vi "Version 1_Read Fullscale Values.vi"(7 "Address (A)":string="A", 8 "error in":errorcluster, 10 "Software version (optional - wire for speed)":u8, 11 "VISA Session In":refnum<visa-resource-name>="Alicat") -> (0 "error out":errorcluster, 1 "Signed?":T1, 2 "Fullscale":T2={"Pressure"=nan, "Volumetric"=nan, "Mass"=nan} {"Pressure" format="%_4f"; "Volumetric" format="%_4f"; "Mass" format="%_4f"}, 3 "VISA Session Out":refnum<visa-resource-name>)   [LabVIEW 2019]
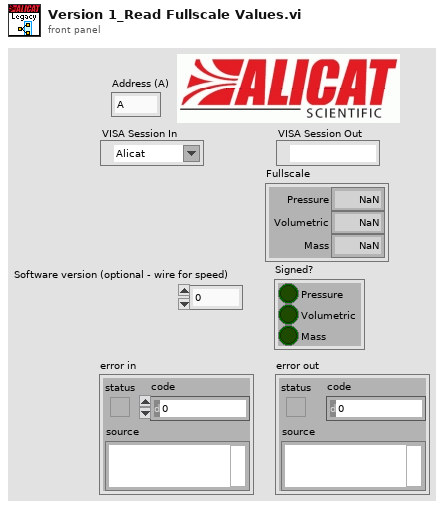
[diagram p1: front panel]
types:
  T1 = cluster{"Pressure":bool, "Volumetric":bool, "Mass":bool}
  T2 = cluster{"Pressure":dbl, "Volumetric":dbl, "Mass":dbl}
  T3 = cluster{"Absolute Pressure":dbl, "Gauge/Diff. Pressure":dbl, "Volumetric Flow":dbl, "Mass Flow":dbl}
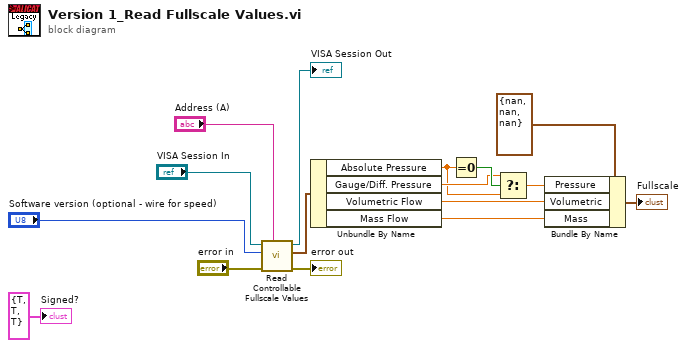
[diagram p0: block diagram]
diagram:
  n1 = call "Read Controllable Fullscale Values.vi"("Unit ID (A)"="Address (A)", "error in"="error in", "Software Version"="Software version (optional - wire for speed)", "VISA Session In"="VISA Session In") -> ("error out"=→"error out":errorcluster, "Fullscale"=w7:T3, "VISA Session Out"=→"VISA Session Out":refnum<visa-resource-name>)  [unwired: 5 in]
  n2 = Unbundle By Name(w7) -> ("Absolute Pressure"=w2:dbl, "Gauge/Diff. Pressure"=w3:dbl, "Volumetric Flow"=w6:dbl, "Mass Flow"=w5:dbl)
  n3 = Equal To 0?(x=w2) -> (x = 0?=w4:bool)
  n4 = Select(t=w3, s=w4, f=w2) -> (s? t:f=w1:dbl)
  n5 = Bundle By Name(cluster=T2 {"Pressure"=nan, "Volumetric"=nan, "Mass"=nan} ("Fullscale"), "Pressure"=w1, "Volumetric"=w6, "Mass"=w5) -> (→"Fullscale":T2)
  "Signed?" <- T1 {"Pressure"=TRUE, "Volumetric"=TRUE, "Mass"=TRUE} ("Signed?")
